vi "slavedone.vi"(9 "index":i32, 11 "shared variable refnum out":refnum<k21>) -> (3 "shared variable refnum out 2":refnum<k21>)   [LabVIEW 2015, in "GageNetwork.lvlib"]
uses:
  Tektronik3102/GageNetwork.lvlib
  Shared program Control/MasterStatus.ctl
  Shared program Control/MySharedVariables.lvlib
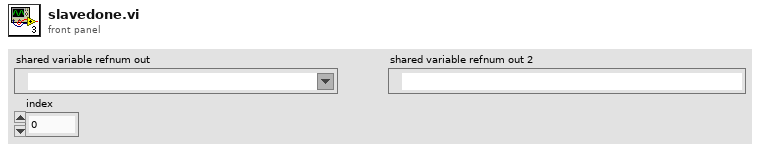
[diagram p1: front panel]
types:
  T1 = typedef "MySharedVariables.lvlib/MasterStatus.ctl" = cluster{"Camera done":bool, "Tektronik done":bool, "Motors done":bool, "Gage":bool}[]
  T2 = cluster{"Camera done":bool, "Tektronik done":bool, "Motors done":bool, "Gage":bool}
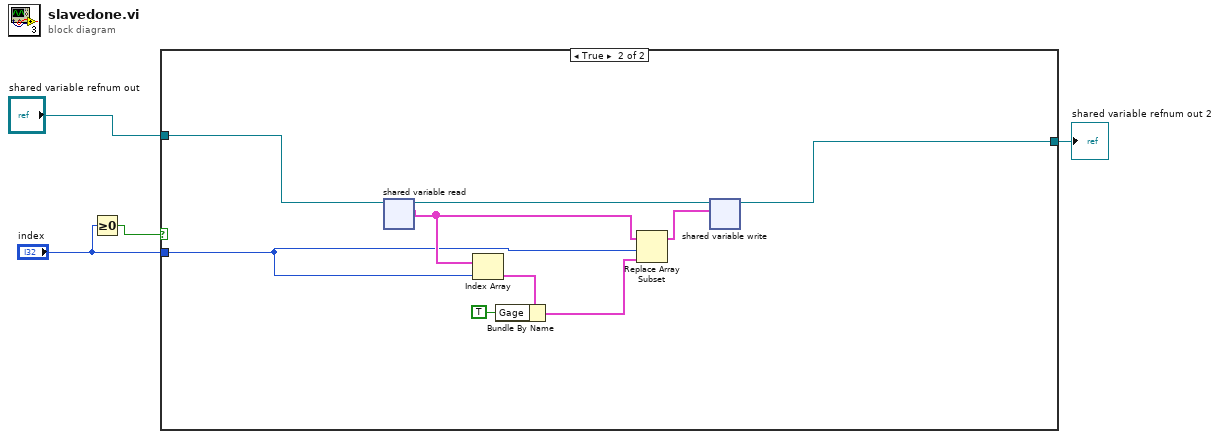
[diagram p0: block diagram]
diagram:
  n1 = Greater Or Equal To 0?(x="index") -> (x >= 0?=w3:bool)
  n2 = case shown="True" w3 {
    tunnel: "index" -> [_ w11]
    tunnel: "shared variable refnum out" -> [w5 w8]
    tunnel: [w5 w7] -> w1
    frame False {
    }
    frame True {
      n3 = shared-variable-read(w8) -> (w14:refnum<k21>, w12:T1)  [unwired: 1 in, 2 out]
      n4 = Index Array(array=w12, index=w11) -> (element=w10:T2)
      n5 = Bundle By Name(cluster=w10, "Gage"=TRUE) -> (w6:T2)
      n6 = Replace Array Subset(array=w12, new element=w6, index=w11) -> (w9:T1)
      n7 = shared-variable-write(w14, w9) -> (w7:refnum<k21>)  [unwired: 1 in, 1 out]
    }
  }
  "shared variable refnum out 2" <- w1
